vi "SetDemMode.vi"(8 "错误输入（无错误）":errorcluster, 11 "检波模式索引值":u8) -> (0 "错误输出":errorcluster)   [LabVIEW 2018]
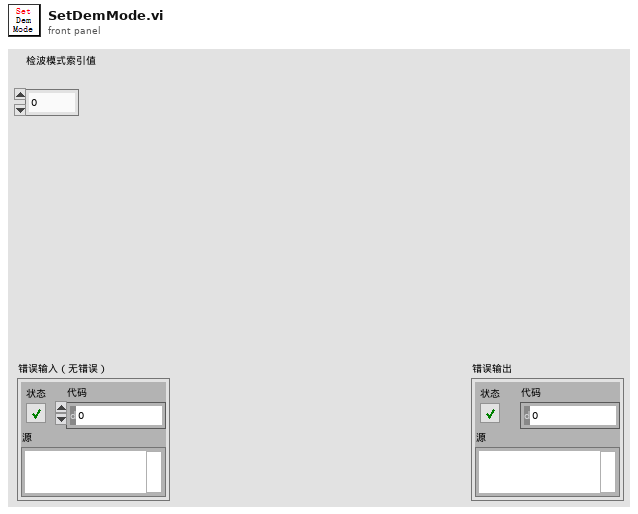
[diagram p1: front panel]
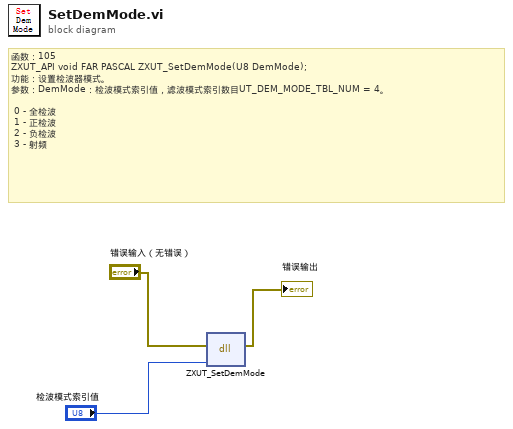
[diagram p0: block diagram]
diagram:
  # "函数：105\nZXUT_API void\tFAR PASCAL ZXUT_SetDemMode(U8 DemMode);\n功能：设置检波器模式。\n参数：DemMode：检波模式索引值，滤波模式索引数目UT_DEM_MODE_TBL_NUM = 4。\n\n\t0 - 全检波\n\t1 - 正检波\n\t2 - 负检波\n\t3 - 射频"
  n1 = dll-call lib="PTH2Rabs E软件项目超声超声子VI函数VI\tTCG处理ZXUTConfigMgr.dll" fn="ZXUT_SetDemMode"(error in="错误输入（无错误）", "DemMode"="检波模式索引值") -> (error out=→"错误输出":errorcluster)  [unwired: 4 in, 1 out]
